vi "CalculatorOperation.vi"(1 "Numeric 2":dbl, 2 "String":string, 3 "Numeric":dbl) -> (0 "Numeric 3":dbl)   [LabVIEW 2015]
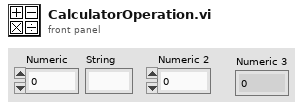
[diagram p1: front panel]
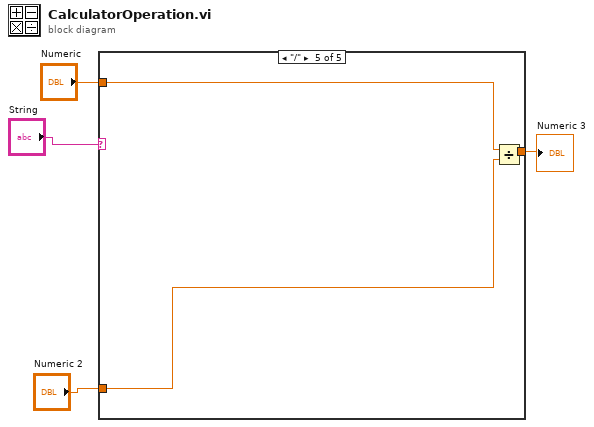
[diagram p0: block diagram]
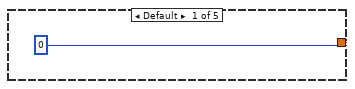
[diagram p2: hidden frame]
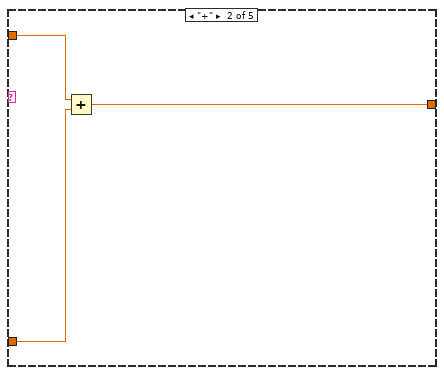
[diagram p3: hidden frame]
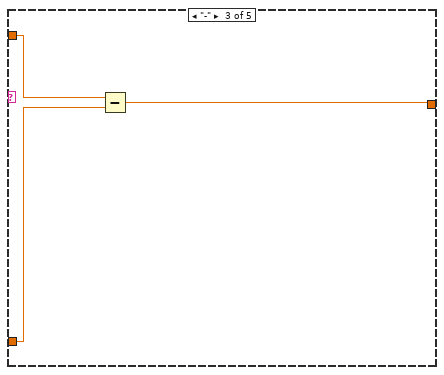
[diagram p4: hidden frame]
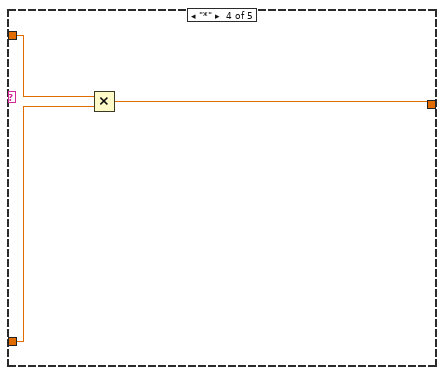
[diagram p5: hidden frame]
diagram:
  n1 = case shown="\"/\"" "String" {
    tunnel: "Numeric" -> [_ w8 w11 w14 w17]
    tunnel: "Numeric 2" -> [_ w7 w10 w13 w15]
    tunnel: [0 w6 w9 w12 w16] -> w1
    frame Default {
    }
    frame "+" {
      n2 = Add(x=w8, y=w7) -> (x+y=w6:dbl)
    }
    frame "-" {
      n3 = Subtract(x=w11, y=w10) -> (x-y=w9:dbl)
    }
    frame "*" {
      n4 = Multiply(x=w14, y=w13) -> (x*y=w12:dbl)
    }
    frame "/" {
      n5 = Divide(x=w17, y=w15) -> (x/y=w16:dbl)
    }
  }
  "Numeric 3" <- w1
